vi "NI VeriStand - Resume Macro Recording.vi"(8 "error in (no error)":errorcluster, 11 "MacroRecorder in":T1) -> (0 "error out":errorcluster, 3 "MacroRecorder out":T1)   [LabVIEW 2020, in "NI_VS MacroRecorderAPI.lvlib"]
doc: "Resumes a stopped macro recording. Use this VI after the Stop Macro Recording VI to append information to the existing macro (.nivsmacro) file in memory."
uses:
  <vilib>/NI VeriStand/Execution/MacroRecorder/NI_VS MacroRecorderAPI.lvlib
  <vilib>/NI VeriStand/Execution/MacroRecorder/MacroRecorderAPI.ctl
  NationalInstruments.VeriStand.ClientAPI
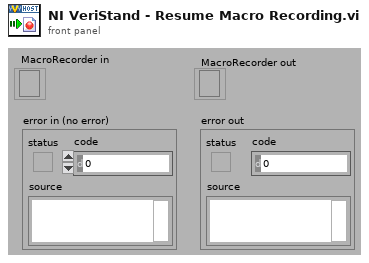
[diagram p1: front panel]
types:
  T1 = typedef "NI_VS MacroRecorderAPI.lvlib/MacroRecorderAPI.ctl" = refnum<k24>
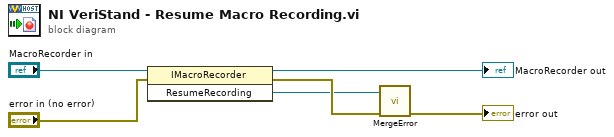
[diagram p0: block diagram]
diagram:
  n1 = invoke class="IMacroRecorder" method="ResumeRecording"(reference="MacroRecorder in", error in="error in (no error)") -> (reference out=→"MacroRecorder out":T1, error out=w4:errorcluster, "ResumeRecording"=w1:refnum<k24>)  [unwired: 1 in]
  n2 = call <vilib>:"MergeError.vi"("error in (no error)"=w4, "Error"=w1) -> ("error out"=→"error out":errorcluster)  [unwired: 9 out]
